vi "lv_mysql_conn_send_command.vi"(8 "error in (no error)":errorcluster, 9 "Message":string, 10 "Command":u8=3 format="%.0x", 11 "connection ID":refnum<k5>) -> (0 "error out":errorcluster, 3 "connection ID out":refnum<k5>)   [LabVIEW 2020]
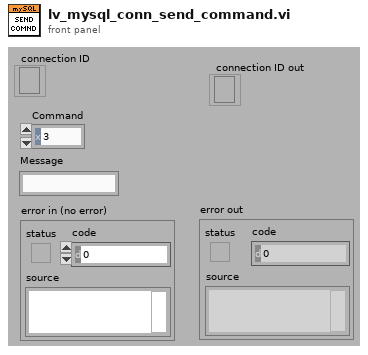
[diagram p1: front panel]
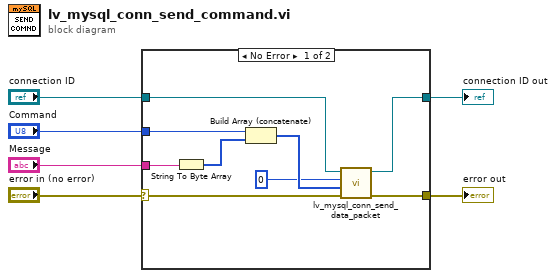
[diagram p0: block diagram]
diagram:
  n1 = case shown="No Error" "error in (no error)" {
    selector: "error in (no error)" -> [w15 w17]
    tunnel: [w14 w17] -> w5
    tunnel: [w12 w16] -> w4
    tunnel: "connection ID" -> [w13 w16]
    tunnel: "Message" -> [w11 _]
    tunnel: "Command" -> [w7 _]
    frame No Error {
      n2 = String To Byte Array(string=w11) -> (unsigned byte array=w10:u8[])
      n3 = Build Array (concatenate)(w7, w10) -> (w9:u8[])
      n4 = call "lv_mysql_conn_send_data_packet.vi"("error in"=w15, "TCP/IP Data"=w9, "Packet #"=u8 0, "connection ID"=w13) -> ("error out"=w14:errorcluster, "connection ID out"=w12:refnum<k5>)  [unwired: 6 in]
    }
    frame Error {
    }
  }
  "error out" <- w5
  "connection ID out" <- w4
